vi "swap_task_lua.vi"(5 "LuaVIEW reference":T1) -> (15 "error out":errorcluster)   [LabVIEW 2012]
doc: "Call the \"Swap Task\" Lua API VI to prepare a new task script and any import scripts. The task with the identifier specified either through the first argument or through the \"--#identifier\" keyword of the script will be signalled to swap the script(s) it is currently executing with the new script(s). This function does not return any run-time errors that occur while the task is swapping.\n\nIf the task script is contained in a file, a relative path or bare filename will be resolved by searching relative to the configured script search directories. If no script search directories are configured, the resource base path is searched. If this function is called from a task context, the directory holding the main script of the calling task is searched first.\nParameters:\nstr:identifier, identifier of the task to swap. When an empty string is specified, an identifier must be provided via the \"--#identifier\" pre-processor keyword.\nstr:name, when the optional task script string is not specified, this is the filename plus any path from which to load the task script. Otherwise it is the name used to refer to the task script when reporting errors.\n[str:script], optional task script string allows direct specification of a bit of Lua code.\nErrors:\nCould not load task script or import script.\nCompilation error in task script or import script.\nError while preprrocessing task script or import script.\nNo task with the specified identifier exists.\nTask does not allow the swap signal."
uses:
  typedefs/t_LuaVIEW Reference.ctl
  subvis/private/LuaVIEW Pull (string).vi
  subvis/private/LuaVIEW Pull (path).vi
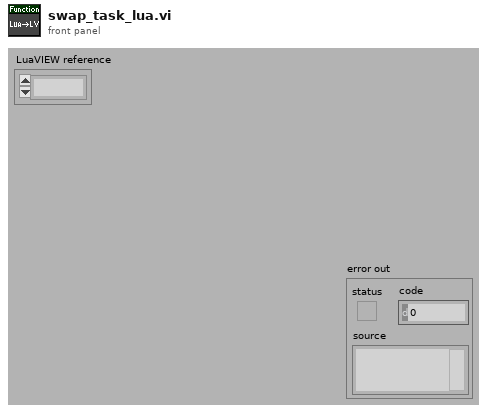
[diagram p1: front panel]
types:
  T1 = typedef "t_LuaVIEW Reference.ctl" = refnum<k1>
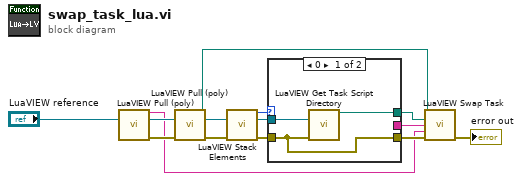
[diagram p0: block diagram]
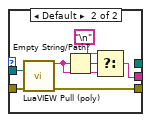
[diagram p2: hidden frame]
diagram:
  n1 = call-poly "LuaVIEW Pull (poly).vi"("LuaVIEW reference in"="LuaVIEW reference") -> ("string"=w1:string, "LuaVIEW reference out"=w3:T1, "error out"=w4:errorcluster)  [unwired: 12 in]
  n2 = call-poly "LuaVIEW Pull (poly).vi"("LuaVIEW reference in"=w3, "error in (no error)"=w4) -> ("path"=w5:path, "LuaVIEW reference out"=w13:T1, "error out"=w14:errorcluster)  [unwired: 11 in]
  n3 = call "LuaVIEW Stack Elements.vi"("LuaVIEW reference in"=w13, "error in (no error)"=w14) -> ("elements"=w12:i32, "LuaVIEW reference out"=w9:T1, "error out"=w11:errorcluster)  [unwired: 11 in]
  n4 = case shown="0" w12 {
    tunnel: w11 -> [w17 w24]
    tunnel: [w17 w23] -> w7
    tunnel: [_ w22] -> w10
    tunnel: w9 -> [w15 w18]
    tunnel: [w16 _] -> w8
    frame 0 {
      n5 = call "LuaVIEW Get Task Script Directory.vi"("LuaVIEW reference in"=w15, "error in (no error)"=w17) -> ("task script directory"=w16:path)  [unwired: 11 in, 2 out]
    }
    frame Default {
      n6 = call-poly "LuaVIEW Pull (poly).vi"("LuaVIEW reference in"=w18, "error in (no error)"=w24) -> ("string"=w20:string, "error out"=w23:errorcluster)  [unwired: 11 in, 1 out]
      n7 = Empty String/Path?(string/path=w20) -> (empty?=w21:bool)
      n8 = Select(t="\n", s=w21, f=w20) -> (s? t:f=w22:string)
    }
  }
  n9 = call "LuaVIEW Swap Task.vi"("script file or name (no name)"=w5, "custom search directory (none)"=w8, "script string (\"\" == load from file)"=w10, "identifier (use keyword)"=w1, "error in (no error)"=w7) -> ("error out"=→"error out":errorcluster)  [unwired: 9 in, 1 out]
